vi "ClearROI.vi"(8 "error in (no error)":errorcluster, 11 "Camera in":refnum<class "Camera.lvclass">) -> (0 "error out":errorcluster, 3 "Camera out":refnum<class "Camera.lvclass">)   [LabVIEW 2020, in "Camera.lvlib" / "Camera.lvclass"]
uses:
  Camera.lvclass
  Camera.lvclass/Camera.ctl
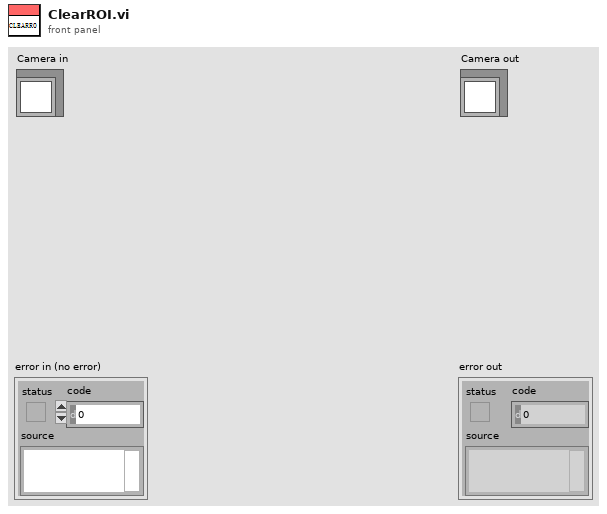
[diagram p1: front panel]
types:
  T1 = typedef "ROI.ctl" = cluster{"x":dbl, "y":dbl, "width":dbl, "height":dbl}
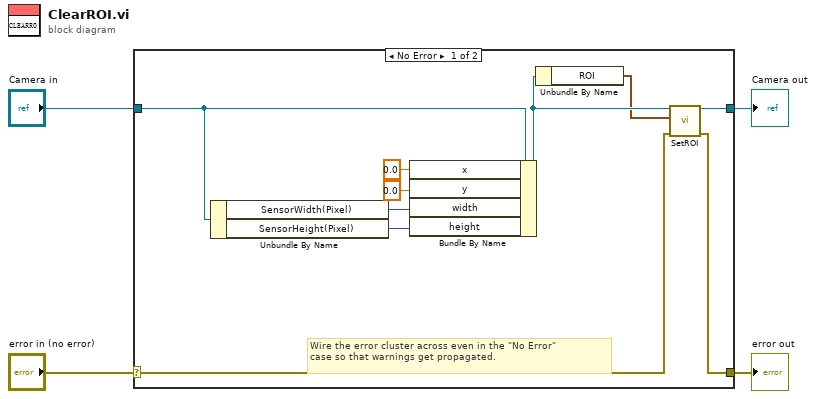
[diagram p0: block diagram]
diagram:
  n1 = case shown="No Error" "error in (no error)" {
    selector: "error in (no error)" -> [w8 w16]
    tunnel: [w7 w16] -> w3
    tunnel: [w9 w15] -> w1
    tunnel: "Camera in" -> [w12 w15]
    frame No Error {
      # "Wire the error cluster across even in the \"No Error\"\ncase so that warnings get propagated."
      n2 = Unbundle By Name(w12) -> ("SensorWidth(Pixel)"=w11:i32, "SensorHeight(Pixel)"=w10:i32)
      n3 = Bundle By Name(cluster=w12, "x"=0.0 ("Setting.ROI.x"), "y"=0.0 ("Setting.ROI.y"), "width"=w11, "height"=w10) -> (w6:refnum<class "Camera.lvclass">)
      n4 = Unbundle By Name(w6) -> ("ROI"=w5:T1)
      n5 = call-dynamic "SetROI.vi"("error in (no error)"=w8, "Setting.ROI"=w5, "Camera in"=w6) -> ("error out"=w7:errorcluster, "Camera out"=w9:refnum<class "Camera.lvclass">)  [unwired: 7 in]
    }
    frame Error {
    }
  }
  "error out" <- w3
  "Camera out" <- w1
